vi "CreateLogStartNode.vi"(7 "DOM Document":refnum<k20>, 8 "Error In":errorcluster, 11 "Log Start Configuration":T1={"Trigger Type"=enum."User", "Timer (sec)"=0.0, "Digital IO Line"=1, "Digital IO Edge"=enum."Rising"}) -> (0 "Error Out":errorcluster, 3 "Start Node":refnum<k20>)   [LabVIEW 2012]
uses:
  LogStartConfiguration.ctl
  LogStartTriggerType.ctl
  LogDigitalIOTriggerEdge.ctl
  libs/LV-Utilities/LV-Utilities.lvlib
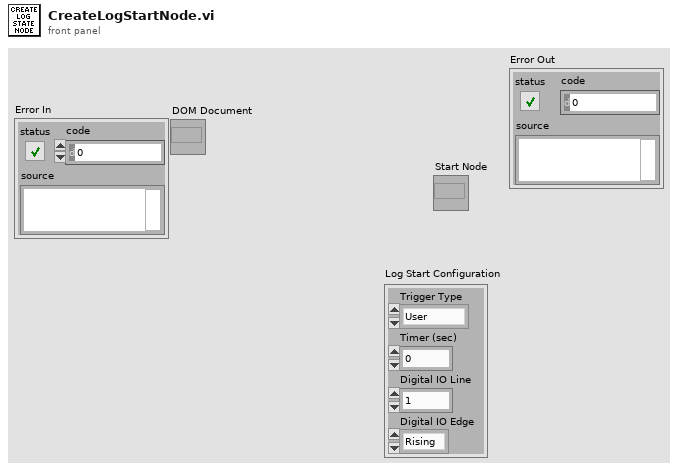
[diagram p1: front panel]
types:
  T1 = typedef "LogStartConfiguration.ctl" = cluster{"Trigger Type":T2, "Timer (sec)":dbl, "Digital IO Line":u8, "Digital IO Edge":T3}
  T2 = typedef "LogStartTriggerType.ctl" = enum16{"Immediate", "User", "Timer", "Digital IO"}
  T3 = typedef "LogDigitalIOTriggerEdge.ctl" = enum16{"Rising", "Falling"}
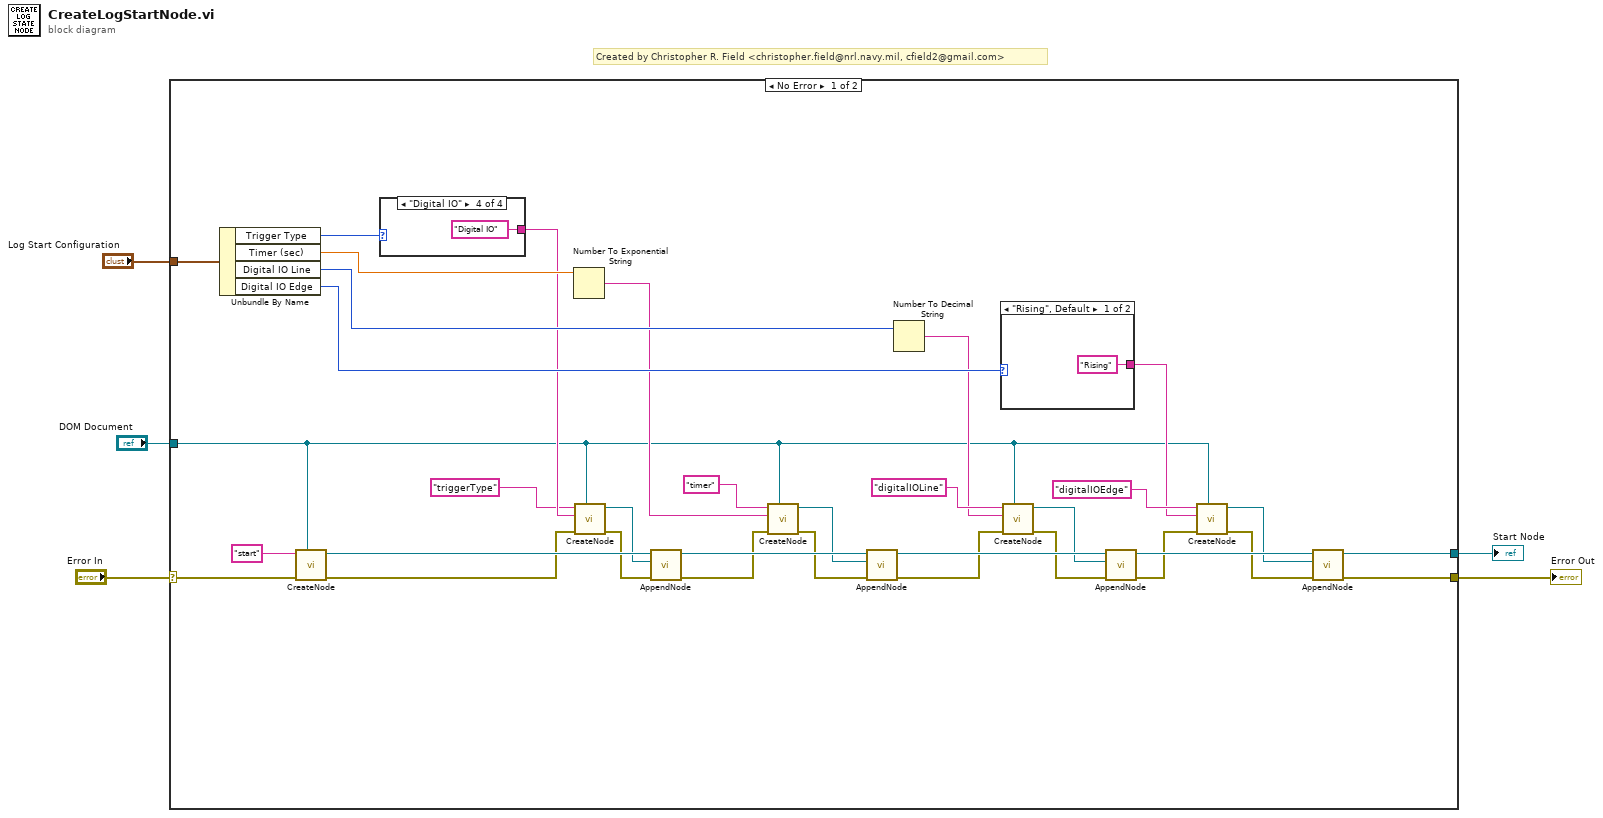
[diagram p0: block diagram]
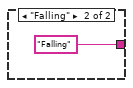
[diagram p2: hidden frame]
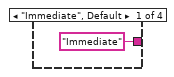
[diagram p3: hidden frame]
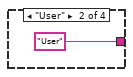
[diagram p4: hidden frame]
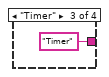
[diagram p5: hidden frame]
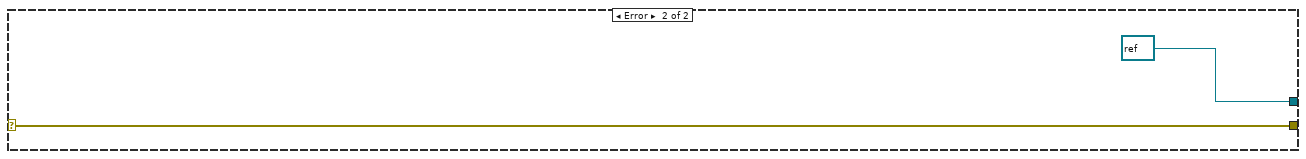
[diagram p6: hidden frame]
diagram:
  # "Created by Christopher R. Field <christopher.field@nrl.navy.mil, cfield2@gmail.com>"
  n1 = case shown="No Error" "Error In" {
    selector: "Error In" -> [w25 w47]
    tunnel: "DOM Document" -> [w6 _]
    tunnel: [w20 refnum<k20> refnum ("Wirings Node 2")] -> w3
    tunnel: [w19 w47] -> w2
    tunnel: "Log Start Configuration" -> [w39 _]
    frame No Error {
      n2 = Unbundle By Name(w39) -> ("Trigger Type"=w38:T2, "Timer (sec)"=w37:dbl, "Digital IO Line"=w36:u8, "Digital IO Edge"=w35:T3)
      n3 = call "CreateNode.vi"("DOM Document"=w6, "Error In"=w25, "Tag Name"="start") -> ("Error out"=w18:errorcluster, "Node"=w24:refnum<k20>)  [unwired: 7 in]
      n4 = case shown="\"Digital IO\"" w38 {
        tunnel: ["Immediate" "User" "Timer" "Digital IO"] -> w34
        frame "Immediate", Default {
        }
        frame "User" {
        }
        frame "Timer" {
        }
        frame "Digital IO" {
        }
      }
      n5 = Number To Exponential String(number=w37) -> (E-format string=w27:string)  [unwired: 3 in]
      n6 = call "CreateNode.vi"("DOM Document"=w6, "Error In"=w18, "Text"=w34, "Tag Name"="triggerType") -> ("Error out"=w17:errorcluster, "Node"=w16:refnum<k20>)  [unwired: 6 in]
      n7 = call "AppendNode.vi"("Error In"=w17, "Child Node"=w16, "Parent Node In"=w24) -> ("Error Out"=w15:errorcluster, "Parent Node Out"=w23:refnum<k20>)  [unwired: 7 in]
      n8 = call "CreateNode.vi"("DOM Document"=w6, "Error In"=w15, "Text"=w27, "Tag Name"="timer") -> ("Error out"=w14:errorcluster, "Node"=w13:refnum<k20>)  [unwired: 6 in]
      n9 = call "AppendNode.vi"("Error In"=w14, "Child Node"=w13, "Parent Node In"=w23) -> ("Error Out"=w12:errorcluster, "Parent Node Out"=w22:refnum<k20>)  [unwired: 7 in]
      n10 = Number To Decimal String(number=w36) -> (decimal integer string=w28:string)  [unwired: 1 in]
      n11 = case shown="\"Rising\", Default" w35 {
        tunnel: ["Rising" "Falling"] -> w29
        frame "Rising", Default {
        }
        frame "Falling" {
        }
      }
      n12 = call "CreateNode.vi"("DOM Document"=w6, "Error In"=w12, "Text"=w28, "Tag Name"="digitalIOLine" ("Text")) -> ("Error out"=w11:errorcluster, "Node"=w8:refnum<k20>)  [unwired: 6 in]
      n13 = call "AppendNode.vi"("Error In"=w11, "Child Node"=w8, "Parent Node In"=w22) -> ("Error Out"=w10:errorcluster, "Parent Node Out"=w21:refnum<k20>)  [unwired: 7 in]
      n14 = call "CreateNode.vi"("DOM Document"=w6, "Error In"=w10, "Text"=w29, "Tag Name"="digitalIOEdge") -> ("Error out"=w9:errorcluster, "Node"=w7:refnum<k20>)  [unwired: 6 in]
      n15 = call "AppendNode.vi"("Error In"=w9, "Child Node"=w7, "Parent Node In"=w21) -> ("Error Out"=w19:errorcluster, "Parent Node Out"=w20:refnum<k20>)  [unwired: 7 in]
    }
    frame Error {
    }
  }
  "Start Node" <- w3
  "Error Out" <- w2
